vi "Kaelus PIM Preset.vi"(7 "Comm Interface":T9, 8 "error in (no error)":errorcluster, 11 "DUT Port (Port 1)":T7) -> (0 "error out":errorcluster, 2 "Flattened TestSetDef w/Version":string, 3 "TestSetDef":T10={"General"={"ID"=0, "Model"="", "Dual Port?"=FALSE, "Options"="", "Options"={"E"=FALSE, "K"=FALSE, "H"=FALSE, "W"=FALSE, "F"=FALSE}, "Cal File"=path ""}, "Receiver"={"Fstart, MHz"=0.0, "Fstop MHz"=0.0, "Fstep MHz"=0.0, "IF, MHz"=0.0}, "RX Band"={"Fstart, MHz"=0.0, "Fstop MHz"=0.0}, "TX 1"={"Fstart, MHz"=0.0, "Fstop MHz"=0.0, "Pmax, dBm"=0.0, "Pstep, dB"=0.0}, "TX 2"={"Fstart, MHz"=0.0, "Fstop MHz"=0.0, "Pmax, dBm"=0.0, "Pstep, dB"=0.0}, "Low-side?"=TRUE})   [LabVIEW 2011]
uses:
  SI.LIB/PIM.LIB/HW IO/Test Set Definition.ctl
  SI.LIB/PIM.LIB/HW IO/DUTport.ctl
  PIM Interface Language.ctl
  PIM Stimulus.ctl
  PIM Cmd Params.ctl
  SI.LIB/PIM.LIB/HW IO/IMOrder.ctl
  SI.LIB/PIM.LIB/HW IO/HW Averaging.ctl
  SI.LIB/PIM.LIB/HW IO/MeasMode.ctl
  SI.LIB/PIM.LIB/DISPLAY/display_unit_format.ctl
  SI.LIB/PIM.LIB/HW IO/PIM Sweep Step Size.ctl
  Kaelus PIM Version.vi
panel:
  out "output cluster":T1={"Carrier Frequencies"={"C1 Freq, MHz"=0.0, "C2 Freq, MHz"=0.0}, "Carrier Powers"={"C1 Power,dBm"=0.0, "C2 Power, dBm"=0.0}, "Measurement Parameters"={"IM Order"=0, "Averaging"=1, "Direction"=0, "Enable ALC?"=FALSE, "Enable SingleIM?"=FALSE, "Display Units"=enum."dBm", "VA Hold?"=FALSE, "DUT PORT"=enum."Port 1"}, "Measurement Setup"={"Meas Type"=enum."Time", "TXStep"=0}} {"Measurement Setup"."TXStep" items=[".2", ".4", "1.0", "2.0"]; "Measurement Parameters"."Direction" items=["Reverse", "Forward", "Auxiliary"]; "Measurement Parameters"."IM Order" items=["3rd", "5th", "7th", "9th", "11th", "13th", "15th", "17th", "19th", "21st", "23rd", "25th", "27th", "29th", "31st", "33rd"]; "Measurement Parameters"."Averaging" items=["None", "Minimum", "Normal", "High", "Maximum"]}
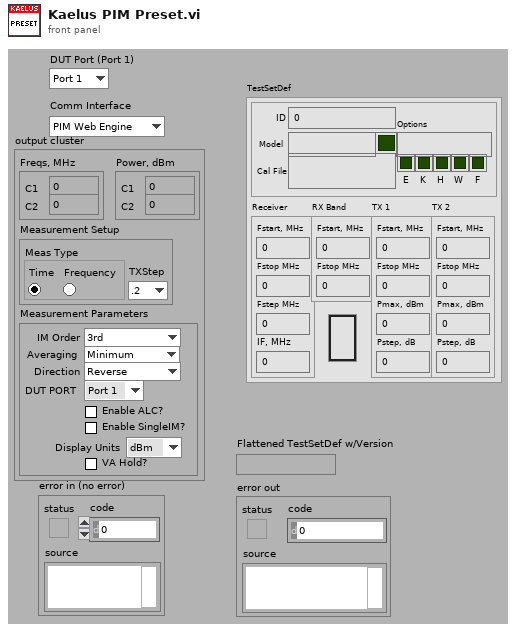
[diagram p1: front panel]
types:
  T1 = typedef "PIM Stimulus.ctl" = cluster{"Carrier Frequencies":cluster{"C1 Freq, MHz":dbl, "C2 Freq, MHz":dbl}, "Carrier Powers":cluster{"C1 Power,dBm":dbl, "C2 Power, dBm":dbl}, "Measurement Parameters":T2, "Measurement Setup":cluster{"Meas Type":enum32{"Time", "Frequency"}, "TXStep":T8}}
  T2 = typedef "PIM Cmd Params.ctl" = cluster{"IM Order":T3, "Averaging":T4, "Direction":T5, "Enable ALC?":bool, "Enable SingleIM?":bool, "Display Units":T6, "VA Hold?":bool, "DUT PORT":T7}
  T3 = typedef "IMOrder.ctl" = u8
  T4 = typedef "HW Averaging.ctl" = u16
  T5 = typedef "MeasMode.ctl" = u16
  T6 = typedef "display_unit_format.ctl" = enum16{"dBm", "dBc"}
  T7 = typedef "DUTport.ctl" = enum16{"Port 1", "Port 2"}
  T8 = typedef "PIM Sweep Step Size.ctl" = u16
  T9 = typedef "PIM Interface Language.ctl" = enum16{"PIM Web Engine", "PIM HW Engine"}
  T10 = typedef "Test Set Definition.ctl" = cluster{"General":cluster{"ID":u32, "Model":string, "Dual Port?":bool, "Options":string, "Options":cluster{"E":bool, "K":bool, "H":bool, "W":bool, "F":bool}, "Cal File":path}, "Receiver":cluster{"Fstart, MHz":dbl, "Fstop MHz":dbl, "Fstep MHz":dbl, "IF, MHz":dbl}, "RX Band":cluster{"Fstart, MHz":dbl, "Fstop MHz":dbl}, "TX 1":cluster{"Fstart, MHz":dbl, "Fstop MHz":dbl, "Pmax, dBm":dbl, "Pstep, dB":dbl}, "TX 2":cluster{"Fstart, MHz":dbl, "Fstop MHz":dbl, "Pmax, dBm":dbl, "Pstep, dB":dbl}, "Low-side?":bool}
  T11 = typedef "OGAB Version.ctl" = cluster{"Version":string, "Build Number":u32, "Build Date/Time":dbl}
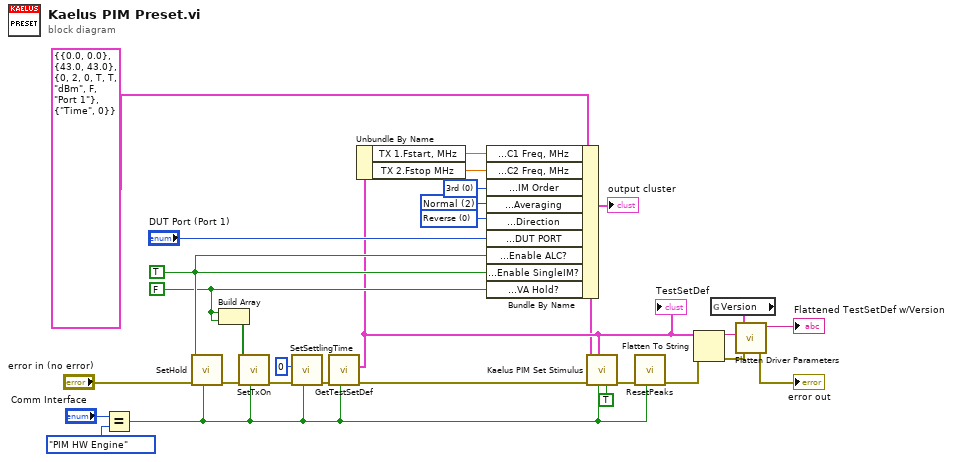
[diagram p0: block diagram]
diagram:
  w18 = FALSE ("VAHold")
  w27 = T3 0 items=["3rd", "5th", "7th", "9th", "11th", "13th", "15th", "17th", "19th", "21st", "23rd", "25th", "27th", "29th", "31st", "33rd"] ("Measurement Parameters.IM Order")
  w26 = T4 2 items=["None", "Minimum", "Normal", "High", "Maximum"] ("Measurement Parameters.Averaging")
  w25 = T5 0 items=["Reverse", "Forward", "Auxiliary"] ("Measurement Parameters.Direction")
  w24 = TRUE ("Measurement Parameters.Enable SingleIM?")
  n1 = Equal?(x="Comm Interface", y=PIM_Interface_Language."PIM HW Engine" ("Interface")) -> (x = y?=w7:bool)
  n2 = call "SetHold.vi"("Legacy (f)?"=w7, "error in (no error)"="error in (no error)", "Hold"=w24) -> ("error out"=w23:errorcluster)  [unwired: 8 out]
  n3 = Build Array(w18, w18) -> (w22:bool[])
  n4 = call "SetTxOn.vi"("Legacy (f)?"=w7, "error in (no error)"=w23, "TxOn"=w22) -> ("error out"=w21:errorcluster)  [unwired: 8 out]
  n5 = call "SetSettlingTime.vi"("Legacy (f)?"=w7, "error in (no error)"=w21, "SettlingTime"=u32 0) -> ("error out"=w5:errorcluster)  [unwired: 8 out]
  n6 = call "GetTestSetDef.vi"("Legacy (f)?"=w7, "error in (no error)"=w5) -> ("error out"=w4:errorcluster, "TestSetDef"=w14:T10)  [unwired: 8 out]
  "TestSetDef" <- w14
  n7 = Unbundle By Name(w14) -> ("TX 1.Fstart, MHz"=w28:dbl, "TX 2.Fstop MHz"=w29:dbl)
  n8 = Bundle By Name(cluster=T1 {"Carrier Frequencies"={"C1 Freq, MHz"=0.0, "C2 Freq, MHz"=0.0}, "Carrier Powers"={"C1 Power,dBm"=43.0, "C2 Power, dBm"=43.0}, "Measurement Parameters"={"IM Order"=0, "Averaging"=2, "Direction"=0, "Enable ALC?"=TRUE, "Enable SingleIM?"=TRUE, "Display Units"=enum."dBm", "VA Hold?"=FALSE, "DUT PORT"=enum."Port 1"}, "Measurement Setup"={"Meas Type"=enum."Time", "TXStep"=0}} ("Stimulus"), "Carrier Frequencies.C1 Freq, MHz"=w28, "Carrier Frequencies.C2 Freq, MHz"=w29, "Measurement Parameters.IM Order"=w27, "Measurement Parameters.Averaging"=w26, "Measurement Parameters.Direction"=w25, "Measurement Parameters.DUT PORT"="DUT Port (Port 1)", "Measurement Parameters.Enable ALC?"=w24, "Measurement Parameters.Enable SingleIM?"=w24, "Measurement Parameters.VA Hold?"=w18) -> (w1:T1)
  "output cluster" <- w1
  n9 = call "Kaelus PIM Set Stimulus.vi"("Force? (f)"=TRUE, "Legacy (f)?"=w7, "TestSetDef"=w14, "error in (no error)"=w4, "Stimulus"=w1) -> ("error out"=w19:errorcluster)  [unwired: 6 out]
  n10 = call "ResetPeaks.vi"("Legacy (f)?"=w7, "error in (no error)"=w19) -> ("error out"=w13:errorcluster)  [unwired: 9 out]
  n11 = Flatten To String(anything=w14, error in (no error)=w13) -> (data string=w15:string, error out=w11:errorcluster)  [unwired: 3 out]
  n12 = global read "Kaelus PIM Version.vi" "Version"() -> (w16:T11)
  n13 = call "Flatten Driver Parameters.vi"("error in (no error)"=w11, "Flattened Driver Parameters (\"\")"=w15, "Driver Version"=w16) -> ("error out"=→"error out":errorcluster, "Flattened Driver Parameters with Version"=→"Flattened TestSetDef w/Version":string)  [unwired: 3 out]
